vi "HAB Climber Global.vi"() -> ()   [LabVIEW 2018]
panel:
  out "HAB Retracting limit":bool
  out "HAB Extending limit":bool
  in  "Disable The VI":bool
  in  "Mode":T1(ring)
  in  "State":enum16{"Retracted", "Extended", "Moving", "N/A"}(ring)
  in  "HAB Retract Speed":dbl
  in  "HAB Extend Speed":dbl
  in  "HAB Encoders":dbl
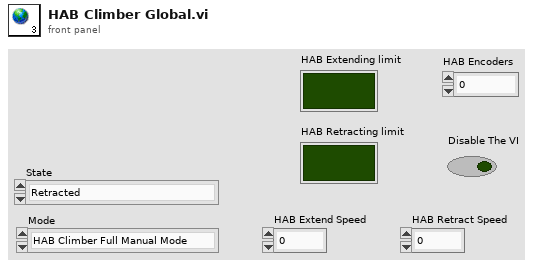
[diagram p1: front panel]
types:
  T1 = enum16{"HAB Climber Full Manual Mode", "HAB Climber Manual Mode", "HAB Climber Automated Mode", "HAB Climber Fully Automated Mode"}
diagram:
